vi "Update Build Versions.vi"(8 "error in (no error)":errorcluster, 11 "PostBuildSupport in":refnum<class "PostBuildSupport.lvclass">) -> (0 "error out":errorcluster, 3 "PostBuildSupport out":refnum<class "PostBuildSupport.lvclass">)   [LabVIEW 2016, in "PostBuildSupport.lvclass"]
uses:
  PostBuildSupport.lvclass
  <vilib>/AppBuilder/AB_API_Simple/Build Specification Version.ctl
  PostBuildSupport.lvclass/PostBuildSupport.ctl
  <vilib>/AppBuilder/AB_API_Simple/Set Build Specification Version (path).vi
  <vilib>/AppBuilder/AB_API_Simple/NI_App_Builder_API.lvlib
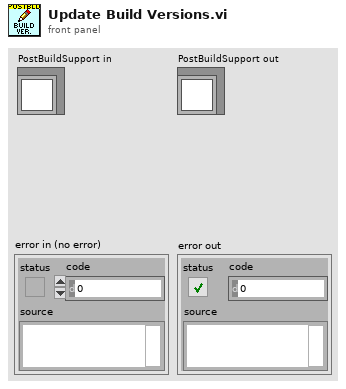
[diagram p1: front panel]
types:
  T1 = typedef "NI_App_Builder_API.lvlib/Build Specification Version.ctl" = cluster{"Major":u16, "Minor":u16, "Fix":u16, "Build":u16}
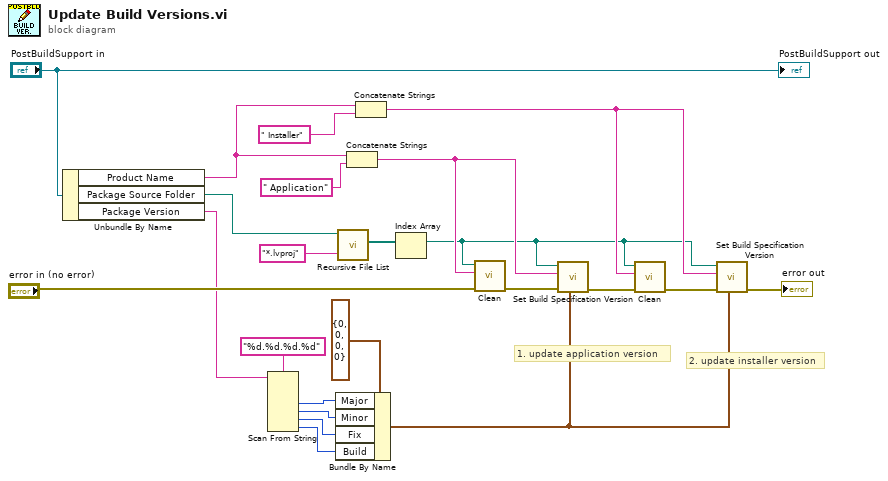
[diagram p0: block diagram]
diagram:
  # "2. update installer version"
  # "1. update application version"
  n1 = Unbundle By Name("PostBuildSupport in") -> ("Product Name"=w2:string, "Package Source Folder"=w3:path, "Package Version"=w1:string)
  n2 = Scan From String(format string="%d.%d.%d.%d", input string=w1) -> (output 1=w18:i32, output 2=w21:i32, output 3=w17:i32, output 4=w20:i32)  [unwired: 6 in, 3 out]
  n3 = Bundle By Name(cluster=T1 {"Major"=0, "Minor"=0, "Fix"=0, "Build"=0} ("Build Specification Version"), "Major"=w18, "Minor"=w21, "Fix"=w17, "Build"=w20) -> (w22:T1)
  n4 = call <vilib>:"Recursive File List.vi"("pattern"="*.lvproj", "Folder Path"=w3) -> ("All Files in Dir"=w6:path[])  [unwired: 5 in, 4 out]
  n5 = Concatenate Strings(w2, " Application" ("Name of target (My Computer)")) -> (w10:string)
  n6 = Concatenate Strings(w2, " Installer" ("Name of target (My Computer)")) -> (w8:string)
  n7 = Index Array(array=w6) -> (element=w5:path)  [unwired: 1 in]
  n8 = call <vilib>:"Clean.vi"("error in (no error)"="error in (no error)", "Name of build specification (if empty: clean all)"=w10, "Path to project"=w5) -> ("error out"=w15:errorcluster)  [unwired: 8 in]
  n9 = call-poly <vilib>:"Set Build Specification Version.vi"("Build Specification Version"=w22, "error in (no error)"=w15, "Name of build specification"=w10, "Path to project"=w5) -> ("error out"=w14:errorcluster)  [unwired: 7 in]
  n10 = call <vilib>:"Clean.vi"("error in (no error)"=w14, "Name of build specification (if empty: clean all)"=w8, "Path to project"=w5) -> ("error out"=w13:errorcluster)  [unwired: 8 in]
  n11 = call-poly <vilib>:"Set Build Specification Version.vi"("Build Specification Version"=w22, "error in (no error)"=w13, "Name of build specification"=w8, "Path to project"=w5) -> ("error out"=→"error out":errorcluster)  [unwired: 7 in]
  "PostBuildSupport out" <- "PostBuildSupport in"
